vi "Get Special Client Paths.vi"(8 "error in":errorcluster, 11 "System in":refnum<class "System.lvclass">) -> (0 "error out":errorcluster, 3 "System out":refnum<class "System.lvclass">)   [LabVIEW 2014, in "System.lvclass"]
uses:
  System.lvclass
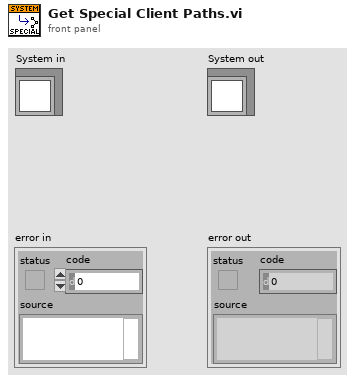
[diagram p1: front panel]
types:
  T1 = typedef "Client Ref.ctl" = cluster{"Name":string, "Path":path}
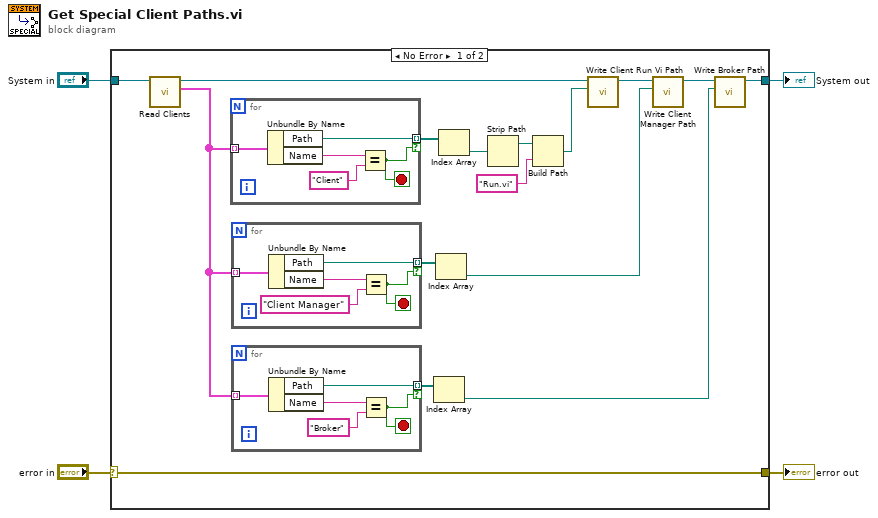
[diagram p0: block diagram]
diagram:
  n1 = case shown="No Error" "error in" {
    selector: "error in" -> [w19 w37]
    tunnel: [w19 w37] -> w3
    tunnel: [w6 w36] -> w1
    tunnel: "System in" -> [w20 w36]
    frame No Error {
      n2 = call-dynamic "Read Clients.vi"("System in"=w20) -> ("Clients"=w8:T1[], "System out"=w18:refnum<class "System.lvclass">)  [unwired: 8 in, 1 out]
      n3 = for {
        tunnel: w8 -> [w35] mode=indexing
        tunnel: [w32] -> w17 mode=indexing if=w31
        stop <- w31 stop-if-true
        n4 = Unbundle By Name(w35) -> ("Path"=w32:path, "Name"=w34:string)
        n5 = Equal?(x=w34, y="Client") -> (x = y?=w31:bool)
      }
      n6 = for {
        tunnel: w8 -> [w30] mode=indexing
        tunnel: [w27] -> w16 mode=indexing if=w26
        stop <- w26 stop-if-true
        n7 = Unbundle By Name(w30) -> ("Path"=w27:path, "Name"=w29:string)
        n8 = Equal?(x=w29, y="Client Manager") -> (x = y?=w26:bool)
      }
      n9 = for {
        tunnel: w8 -> [w25] mode=indexing
        tunnel: [w22] -> w7 mode=indexing if=w21
        stop <- w21 stop-if-true
        n10 = Unbundle By Name(w25) -> ("Path"=w22:path, "Name"=w24:string)
        n11 = Equal?(x=w24, y="Broker") -> (x = y?=w21:bool)
      }
      n12 = Index Array(array=w7) -> (element=w5:path)  [unwired: 1 in]
      n13 = Index Array(array=w16) -> (element=w9:path)  [unwired: 1 in]
      n14 = Index Array(array=w17) -> (element=w13:path)  [unwired: 1 in]
      n15 = Strip Path(path=w13) -> (stripped path=w15:path)  [unwired: 1 out]
      n16 = Build Path(base path=w15, name or relative path="Run.vi" ("Client Name")) -> (appended path=w11:path)
      n17 = call-dynamic "Write Client Run Vi Path.vi"("Client Run Vi Path"=w11, "System in"=w18) -> ("System out"=w12:refnum<class "System.lvclass">)  [unwired: 8 in, 1 out]
      n18 = call-dynamic "Write Client Manager Path.vi"("Client Manager Path"=w9, "System in"=w12) -> ("System out"=w10:refnum<class "System.lvclass">)  [unwired: 8 in, 1 out]
      n19 = call-dynamic "Write Broker Path.vi"("Broker Path"=w5, "System in"=w10) -> ("System out"=w6:refnum<class "System.lvclass">)  [unwired: 8 in, 1 out]
    }
    frame Error {
    }
  }
  "error out" <- w3
  "System out" <- w1
